vi "Actor Core.vi"(8 "error in":errorcluster, 11 "Nested in":refnum<class "ACQ Contador.lvclass">) -> (0 "error out":errorcluster, 3 "Actor out":refnum<class "Actor.lvclass">)   [LabVIEW 2020, in "ACQ Contador.lvlib" / "ACQ Contador.lvclass"]
doc: "(<B>Filename</B>: Actor Framework.lvlib:Actor.lvclass:Actor Core.vi)\n\nReceives messages to the actor, reacts to them, and initiates any error handling that may shut the actor down.\n\nDescendant classes may override this VI to append parallel tasks for the actor to complete while it handles messages. Overrides use the Call Parent Method node."
uses:
  ACQ Contador.lvclass
  C:/Program Files (x86)/National Instruments/LabVIEW 2020/vi.lib/ActorFramework/Actor/Actor.lvclass
  <vilib>/ActorFramework/Actor/Actor.lvclass
  <vilib>/ActorFramework/Actor/Actor.lvclass/Actor.ctl
  ACQ Contador.lvclass/ACQ Contador.ctl
  Contador Messages/Actualiza Contador Msg/Actualiza Contador Msg.lvclass/Actualiza Contador Msg.ctl
  <vilib>/ActorFramework/Message Enqueuer/Message Enqueuer.lvclass/Message Enqueuer.ctl
  <vilib>/ActorFramework/Message Enqueuer/Enqueue.vi
  Contador Messages/Actualiza Contador Msg/Actualiza Contador Msg.lvclass
  C:/Program Files (x86)/National Instruments/LabVIEW 2020/vi.lib/ActorFramework/Message/Message.lvclass
  <vilib>/ActorFramework/Message Priority Queue/Priority Enqueue.vi
types:
  T1 = cluster{"Exit":refnum<user-event>, "Start/Stop":refnum<user-event>, "File Type":refnum<user-event>, "Lim Superior":refnum<user-event>, "Lim Inferior":refnum<user-event>, "Path":refnum<user-event>, "Save Enable":refnum<user-event>}
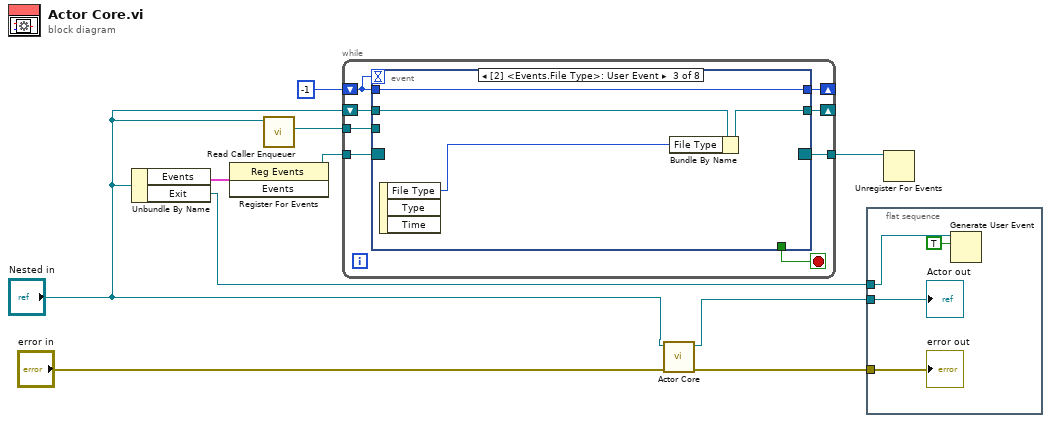
[diagram p0: block diagram]
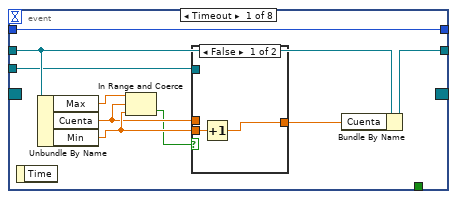
[diagram p2: hidden frame]
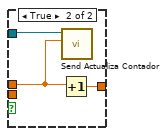
[diagram p3: hidden frame]
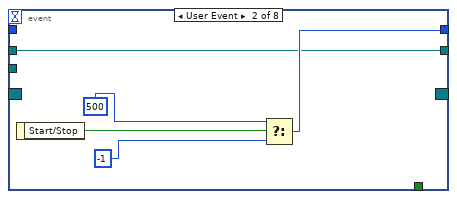
[diagram p4: hidden frame]
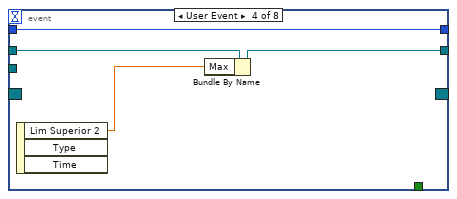
[diagram p5: hidden frame]
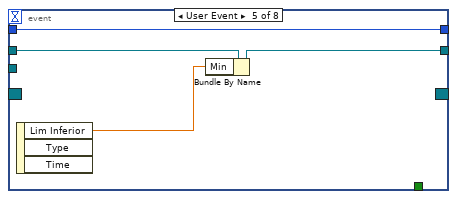
[diagram p6: hidden frame]
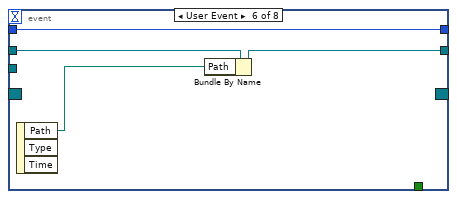
[diagram p7: hidden frame]
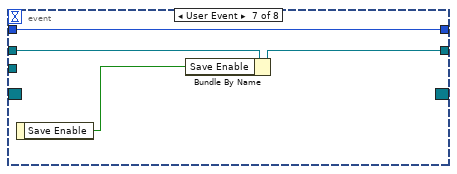
[diagram p8: hidden frame]
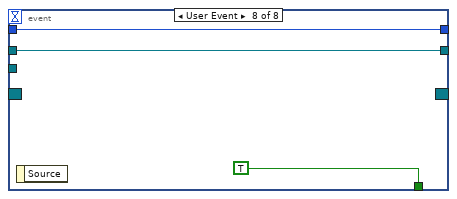
[diagram p9: hidden frame]
diagram:
  n1 = Unbundle By Name("Nested in") -> ("Events"=w10:T1, "Exit"=w9:refnum<user-event>)
  n2 = register-events(w10) -> (reference out=w8:refnum<event-registration>)  [unwired: 2 in, 1 out]
  n3 = call <vilib>:"Read Caller Enqueuer.vi"("Actor"="Nested in") -> ("Caller Enqueuer"=w7:refnum<class "Message Enqueuer.lvclass">)  [unwired: 10 in]
  n4 = while {
    tunnel: w8 -> [w18]
    tunnel: w7 -> [w17]
    tunnel: [w15] -> w6
    shift-right: [w13] -> _
    shift-left: -1 -> [w14]
    shift-right: [w11] -> _
    shift-left: "Nested in" -> [w12]
    stop <- w16 stop-if-true
    n5 = event shown="[2] <Events.File Type>: User Event" {
      selector: w18 -> [_ _ _ _ _ _ _ _]
      dyn-events: [_ _ _ _ _ _ _ _] -> w15
      timeout: w14 -> [_ _ _ _ _ _ _ _]
      tunnel: w17 -> [w24 _ _ _ _ _ _ _]
      tunnel: [_ _ _ _ _ _ _ TRUE] -> w16
      tunnel: w14 -> [w27 _ w41 w45 w49 w53 w57 w59]
      tunnel: [w27 w36 w41 w45 w49 w53 w57 w59] -> w13
      tunnel: w12 -> [w26 w33 w40 w44 w48 w52 w56 w58]
      tunnel: [w25 w33 w39 w43 w47 w51 w55 w58] -> w11
      event Timeout {
        n6 = event-data() -> ()  [unwired: 1 in, 1 out]
        n7 = Unbundle By Name(w26) -> ("Max"=w20:dbl, "Cuenta"=w21:dbl, "Min"=w22:dbl)
        n8 = In Range and Coerce(upper limit=w20, x=w21, lower limit=w22) -> (In Range?=w19:bool)  [unwired: 1 out]
        n9 = case shown="False" w19 {
          tunnel: w21 -> [_ w31]
          tunnel: w24 -> [_ w32]
          tunnel: [w28 w30] -> w23
          tunnel: w22 -> [w29 _]
          frame False {
            n10 = Increment(x=w29) -> (x+1=w28:dbl)
          }
          frame True {
            n11 = Increment(x=w31) -> (x+1=w30:dbl)
            n12 = call "Send Actualiza Contador.vi"("Contador"=w31, "Message Enqueuer"=w32) -> ()  [unwired: 8 in, 2 out]
          }
        }
        n13 = Bundle By Name(cluster=w26, "Cuenta"=w23) -> (w25:refnum<class "ACQ Contador.lvclass">)
      }
      event User Event {
        n14 = event-data() -> ("Start/Stop"=w37:bool)  [unwired: 1 in]
        n15 = Select(t=500, s=w37, f=-1) -> (s? t:f=w36:i32)
      }
      event User Event {
        n16 = event-data() -> ("File Type"=w38:enum16{""})  [unwired: 1 in, 2 out]
        n17 = Bundle By Name(cluster=w40, "File Type"=w38) -> (w39:refnum<class "ACQ Contador.lvclass">)
      }
      event User Event {
        n18 = event-data() -> ("Lim Superior 2"=w42:dbl)  [unwired: 1 in, 2 out]
        n19 = Bundle By Name(cluster=w44, "Max"=w42) -> (w43:refnum<class "ACQ Contador.lvclass">)
      }
      event User Event {
        n20 = event-data() -> ("Lim Inferior"=w46:dbl)  [unwired: 1 in, 2 out]
        n21 = Bundle By Name(cluster=w48, "Min"=w46) -> (w47:refnum<class "ACQ Contador.lvclass">)
      }
      event User Event {
        n22 = event-data() -> ("Path"=w50:path)  [unwired: 1 in, 2 out]
        n23 = Bundle By Name(cluster=w52, "Path"=w50) -> (w51:refnum<class "ACQ Contador.lvclass">)
      }
      event User Event {
        n24 = event-data() -> ("Save Enable"=w54:bool)  [unwired: 1 in]
        n25 = Bundle By Name(cluster=w56, "Save Enable"=w54) -> (w55:refnum<class "ACQ Contador.lvclass">)
      }
      event User Event {
        n26 = event-data() -> ()  [unwired: 1 in, 1 out]
      }
    }
  }
  n27 = call-parent "Actor Core.vi"("error in"="error in", "Actor in"="Nested in") -> ("error out"=w5:errorcluster, "Actor out"=w3:refnum<class "Actor.lvclass">)  [unwired: 8 in]
  n28 = flat-sequence {
    tunnel: w5 -> [w64]
    tunnel: w9 -> [w63]
    tunnel: w3 -> [w61]
    frame #0 {
      n29 = Generate User Event(user event=w63, event data cluster=TRUE ("event data")) -> ()  [unwired: 2 in, 2 out]
      "error out" <- w64
      "Actor out" <- w61
    }
  }
  n30 = Unregister For Events(event registration refnum=w6) -> ()  [unwired: 1 in, 1 out]
